vi "read_avg_traj_pks.vi"(0 "all rows":dbl[][](array[numeric])) -> (4 "Graph":cluster{"Locations":dbl[], "Amplitudes":dbl[]}[](graph), 5 "avg_trajx":dbl[](array[numeric]), 6 "avg_trajy":dbl[](array[numeric]), 7 "avg_trajz":dbl[](array[numeric]), 8 "std_trajz":dbl, 9 "std_trajx":dbl, 10 "std_trajy":dbl)   [LabVIEW 2024]
uses:
  <vilib>/Analysis/NI_AALBase.lvlib
  <vilib>/Analysis/baseanly.llb/Mean (DBL).vi
  <vilib>/Analysis/NI_AAL_SigProc.lvlib
  <vilib>/Analysis/3filter.llb/Butterworth Filter (DBL).vi
panel:
  out "max value":dbl
  out "min value":dbl
  out "subarray":dbl[](array[numeric])
  out "Graph  2":cluster{"avg_trajx":dbl[], "avg_trajz":dbl[]}(graph)
  out "pkavgloctn":dbl[](array[numeric])
  out "largerv":dbl[](array[numeric])
  out "smallerv":dbl[](array[numeric])
  out "locations":i32[](array[numeric])
  out "# found y":i32
  out "# found z":i32
  out "ypkLocations":dbl[](array[numeric])
  out "zpkLocations":dbl[](array[numeric])
  out "z_pelv_center":dbl[](array[numeric])
  out "y_pelv_center":dbl[](array[numeric])
  out "x_pelv_center":dbl[](array[numeric])
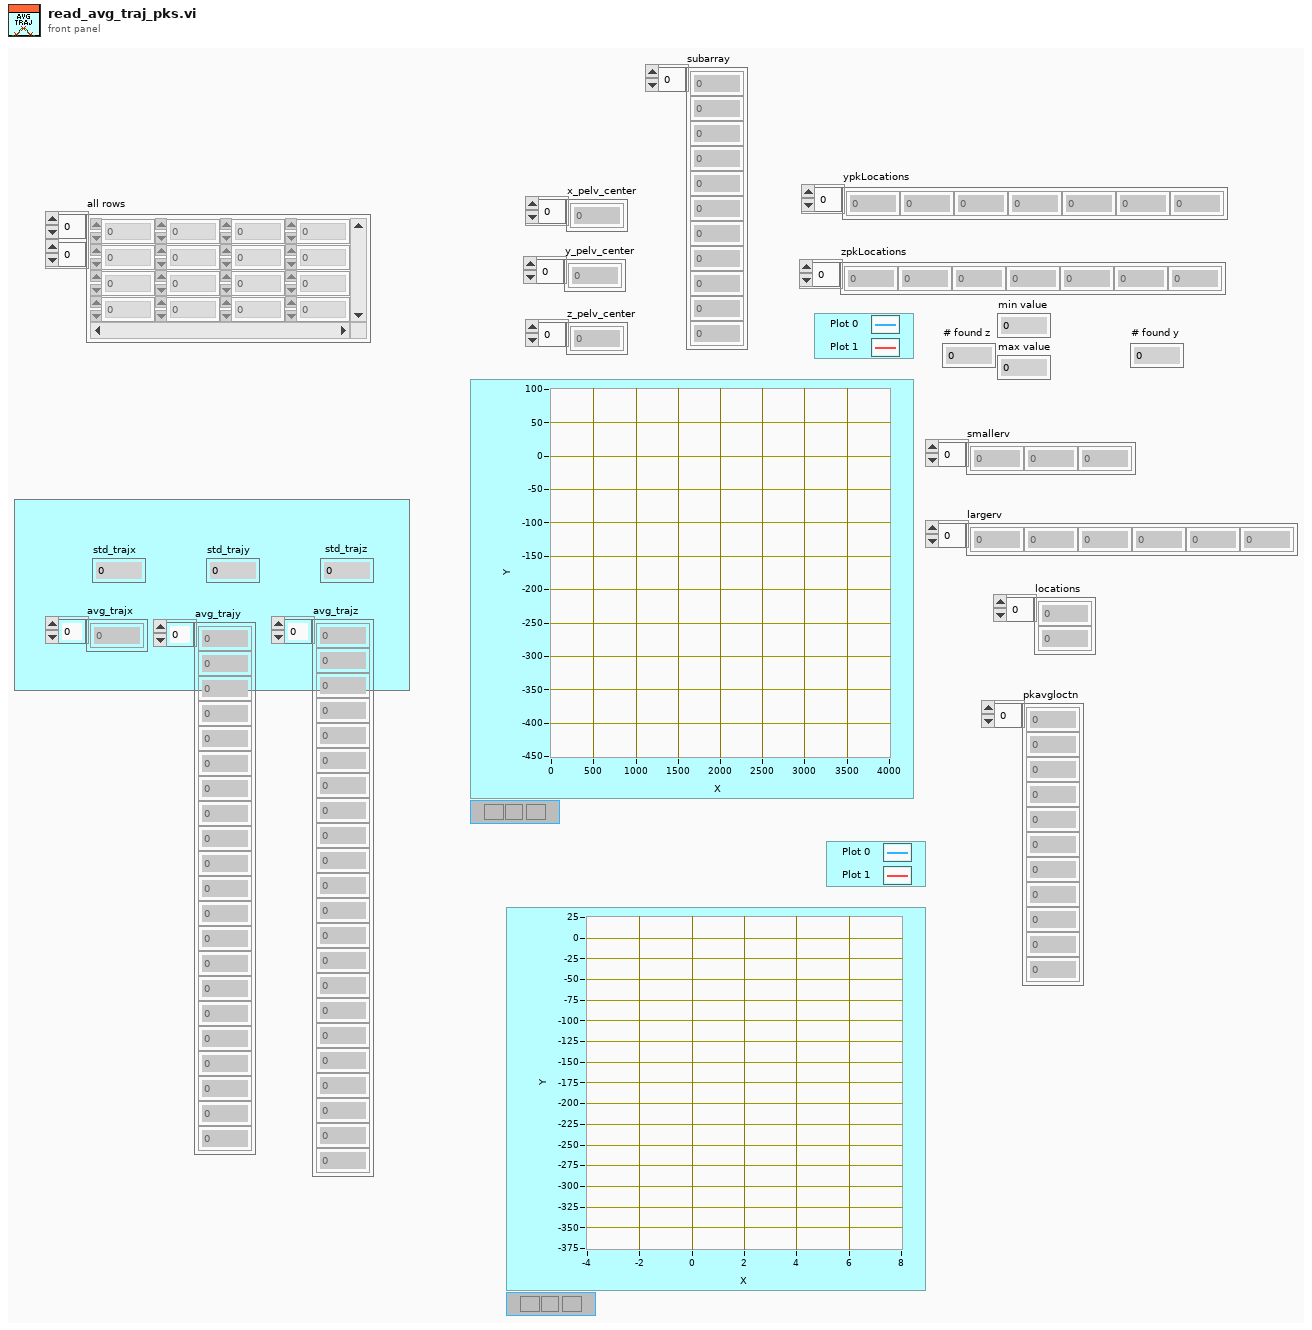
[diagram p1: front panel]
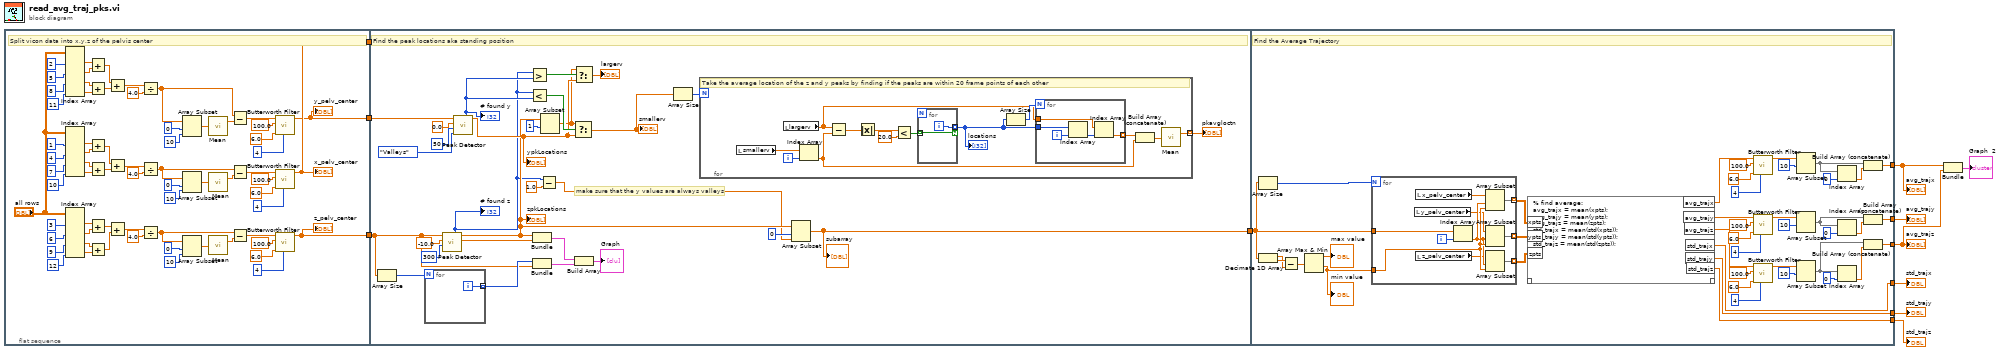
[diagram p0: block diagram]
diagram:
  n1 = flat-sequence {
    tunnel: [w12] -> w11
    tunnel: [w13] -> w10
    tunnel: [w14] -> w9
    tunnel: w11 -> [w80]
    tunnel: w10 -> [w79]
    tunnel: w9 -> [_]
    tunnel: [w81] -> w1
    tunnel: [w134] -> w5
    tunnel: [w137] -> w3
    tunnel: [w162] -> w8
    tunnel: [w129] -> w2
    tunnel: [w161] -> w7
    tunnel: [w160] -> w6
    tunnel: w1 -> [w166]
    frame #0 {
      # "Split vicon data into x,y,z of the pelvis center"
      n2 = Index Array(array="all rows", index (col) #1=2 ("disabled index (col)"), index (col) #2=5 ("index (col)"), index (col) #3=8 ("index (col)"), index (col) #4=11 ("index (col)")) -> (element #1=w59:dbl[], element #2=w58:dbl[], element #3=w57:dbl[], element #4=w56:dbl[])  [unwired: 4 in]
      n3 = Index Array(array="all rows", index (col) #1=1 ("disabled index (col)"), index (col) #2=4 ("index (col)"), index (col) #3=7 ("index (col)"), index (col) #4=10 ("index (col)")) -> (element #1=w72:dbl[], element #2=w71:dbl[], element #3=w70:dbl[], element #4=w69:dbl[])  [unwired: 4 in]
      n4 = Index Array(array="all rows", index (col) #1=3 ("disabled index (col)"), index (col) #2=6 ("index (col)"), index (col) #3=9 ("index (col)"), index (col) #4=12 ("index (col)")) -> (element #1=w46:dbl[], element #2=w45:dbl[], element #3=w44:dbl[], element #4=w43:dbl[])  [unwired: 4 in]
      n5 = Add(x=w59, y=w58) -> (x+y=w61:dbl[])
      n6 = Add(x=w57, y=w56) -> (x+y=w60:dbl[])
      n7 = Add(x=w72, y=w71) -> (x+y=w74:dbl[])
      n8 = Add(x=w70, y=w69) -> (x+y=w73:dbl[])
      n9 = Add(x=w46, y=w45) -> (x+y=w48:dbl[])
      n10 = Add(x=w44, y=w43) -> (x+y=w47:dbl[])
      n11 = Add(x=w61, y=w60) -> (x+y=w54:dbl[])
      n12 = Add(x=w74, y=w73) -> (x+y=w67:dbl[])
      n13 = Add(x=w48, y=w47) -> (x+y=w41:dbl[])
      n14 = Divide(x=w54, y=4.0) -> (x/y=w32:dbl[])
      n15 = Divide(x=w67, y=4.0) -> (x/y=w38:dbl[])
      n16 = Divide(x=w41, y=4.0) -> (x/y=w27:dbl[])
      n17 = Array Subset(array=w32, index=0, length=10) -> (w31:dbl[])
      n18 = Array Subset(array=w38, index=0, length=10) -> (w35:dbl[])
      n19 = Array Subset(array=w27, index=0, length=10) -> (w28:dbl[])
      n20 = call-poly <vilib>:"Mean.vi"("X"=w31) -> ("mean"=w53:dbl)  [unwired: 1 out]
      n21 = call-poly <vilib>:"Mean.vi"("X"=w35) -> ("mean"=w66:dbl)  [unwired: 1 out]
      n22 = call-poly <vilib>:"Mean.vi"("X"=w28) -> ("mean"=w40:dbl)  [unwired: 1 out]
      n23 = Subtract(x=w32, y=w53) -> (x-y=w15:dbl[])
      n24 = Subtract(x=w38, y=w66) -> (x-y=w19:dbl[])
      n25 = Subtract(x=w27, y=w40) -> (x-y=w26:dbl[])
      n26 = call-poly <vilib>:"Butterworth Filter.vi"("order"=4, "low cutoff freq: fl"=6.0, "sampling freq: fs"=100.0, "X"=w15) -> ("Filtered X"=w12:dbl[])  [unwired: 4 in, 1 out]
      "y_pelv_center" <- w12
      n27 = call-poly <vilib>:"Butterworth Filter.vi"("order"=4, "low cutoff freq: fl"=6.0, "sampling freq: fs"=100.0, "X"=w19) -> ("Filtered X"=w14:dbl[])  [unwired: 4 in, 1 out]
      "x_pelv_center" <- w14
      n28 = call-poly <vilib>:"Butterworth Filter.vi"("order"=4, "low cutoff freq: fl"=6.0, "sampling freq: fs"=100.0, "X"=w26) -> ("Filtered X"=w13:dbl[])  [unwired: 4 in, 1 out]
      "z_pelv_center" <- w13
    }
    frame #1 {
      # "make sure that the y values are always valleys"
      # "Find the peak locations aka standing position"
      n29 = Array Size(array=w79) -> (size(s)=w105:i32)
      n30 = for {
        N: w105 -> [_]
        tunnel: [w128] -> w101 mode=indexing
        i -> [w128]
      }
      n31 = call <vilib>:"Peak Detector.vi"("width"=300, "threshold"=-10.0, "X"=w79) -> ("Amplitudes"=w106:dbl[], "Locations"=w86:dbl[], "# found"=w83:i32)  [unwired: 4 in, 2 out]
      "zpkLocations" <- w86
      "# found z" <- w83
      n32 = call <vilib>:"Peak Detector.vi"("peaks/valleys"=enum32{"Peaks", "Valleys"}."Valleys", "width"=50, "threshold"=0.0, "X"=w80) -> ("Locations"=w95:dbl[], "# found"=w97:i32)  [unwired: 3 in, 3 out]
      "ypkLocations" <- w95
      "# found y" <- w97
      n33 = Greater?(x=w83, y=w97) -> (0:w96:bool)
      n34 = Less?(x=w83, y=w97) -> (x < y?=w98:bool)
      n35 = Bundle("Locations"=w86, "Amplitudes"=w106) -> (w104:cluster{"Locations":dbl[], "Amplitudes":dbl[]})  [unwired: 1 in]
      n36 = Bundle(w101, "Filtered X"=w79) -> (w102:cluster{i32[], "Filtered X":dbl[]})  [unwired: 1 in]
      n37 = Subtract(x=w83, y=1.0) -> (x-y=w82:dbl)
      n38 = Array Subset(array=w86, index=1) -> (w88:dbl[])  [unwired: 1 in]
      n39 = Select(t=w88, s=w98, f=w95) -> (s? t:f=w94:dbl[])
      "smallerv" <- w94
      n40 = Select(t=w88, s=w96, f=w95) -> (s? t:f=→"largerv":dbl[])
      n41 = Build Array(w104, w102) -> (→"Graph":cluster{"Locations":dbl[], "Filtered X":dbl[]}[])
      n42 = Array Size(array=w94) -> (size(s)=w92:i32)
      n43 = for {
        N: w92 -> [_]
        tunnel: [w108] -> w87 mode=indexing
        i -> [w120]
        # "Take the average location of the z and y peaks by finding if the peaks are within 20 frame points of each other"
        n44 = local read "smallerv"() -> (w119:dbl[])
        n45 = local read "largerv"() -> (w113:dbl[])
        n46 = Index Array(array=w119, index=w120) -> (element=w110:dbl)
        n47 = Subtract(x=w113, y=w110) -> (x-y=w116:dbl[])
        n48 = Absolute Value(x=w116) -> (abs(x)=w117:dbl[])
        n49 = Less?(x=w117, y=20.0) -> (x < y?=w118:bool[])
        n50 = for {
          tunnel: w118 -> [w127] mode=indexing
          tunnel: [w126] -> w112 mode=indexing if=w127
          i -> [w126]
        }
        "locations" <- w112
        n51 = Array Size(array=w112) -> (size(s)=w114:i32)
        n52 = for {
          N: w114 -> [_]
          tunnel: w113 -> [w125]
          tunnel: w112 -> [w123]
          tunnel: [w121] -> w111 mode=indexing
          i -> [w124]
          n53 = Index Array(array=w123, index=w124) -> (element=w122:i32)
          n54 = Index Array(array=w125, index=w122) -> (element=w121:dbl)
        }
        n55 = Build Array (concatenate)(w111, w110) -> (w109:dbl[])
        n56 = call-poly <vilib>:"Mean.vi"("X"=w109) -> ("mean"=w108:dbl)  [unwired: 1 out]
      }
      "pkavgloctn" <- w87
      n57 = Array Subset(array=w86, index=0, length=w82) -> (w81:dbl[])
      "subarray" <- w81
    }
    frame #2 {
      # "Find the Average Trajectory"
      n58 = Array Size(array=w166) -> (size(s)=w168:i32)
      n59 = Decimate 1D Array(w166) -> (w170:dbl[], w171:dbl[])
      n60 = Subtract(x=w171, y=w170) -> (x-y=w169:dbl[])
      n61 = Array Max & Min(array=w169) -> (max value=→"max value":dbl, min value=w167:dbl)  [unwired: 2 out]
      "min value" <- w167
      n62 = for {
        N: w168 -> [_]
        tunnel: w167 -> [w181]
        tunnel: w166 -> [w180]
        tunnel: [w174] -> w165 mode=indexing
        tunnel: [w173] -> w164 mode=indexing
        tunnel: [w172] -> w163 mode=indexing
        i -> [w179]
        n63 = local read "y_pelv_center"() -> (w176:dbl[])
        n64 = local read "x_pelv_center"() -> (w177:dbl[])
        n65 = local read "z_pelv_center"() -> (w175:dbl[])
        n66 = Index Array(array=w180, index=w179) -> (element=w178:dbl)
        n67 = Array Subset(array=w177, index=w178, length=w181) -> (w174:dbl[])
        n68 = Array Subset(array=w176, index=w178, length=w181) -> (w173:dbl[])
        n69 = Array Subset(array=w175, index=w178, length=w181) -> (w172:dbl[])
      }
      n70 = mathscript code="% find average:\navg_trajx = mean(xpts);\navg_trajy = mean(ypts);\navg_trajz = mean(zpts);\nstd_trajx = mean(std(xpts));\nstd_trajy = mean(std(ypts));\nstd_trajz = mean(std(zpts));"("xpts"=w165, "ypts"=w164, "zpts"=w163) -> ("avg_trajx"=w156:dbl[], "avg_trajy"=w152:dbl[], "avg_trajz"=w148:dbl[], "std_trajx"=w160:dbl, "std_trajy"=w162:dbl, "std_trajz"=w161:dbl)  [unwired: 1 in, 1 out]
      n71 = call-poly <vilib>:"Butterworth Filter.vi"("order"=4, "low cutoff freq: fl"=6.0, "sampling freq: fs"=100.0, "X"=w156) -> ("Filtered X"=w146:dbl[])  [unwired: 4 in, 1 out]
      n72 = call-poly <vilib>:"Butterworth Filter.vi"("order"=4, "low cutoff freq: fl"=6.0, "sampling freq: fs"=100.0, "X"=w152) -> ("Filtered X"=w144:dbl[])  [unwired: 4 in, 1 out]
      n73 = call-poly <vilib>:"Butterworth Filter.vi"("order"=4, "low cutoff freq: fl"=6.0, "sampling freq: fs"=100.0, "X"=w148) -> ("Filtered X"=w142:dbl[])  [unwired: 4 in, 1 out]
      n74 = Array Subset(array=w146, index=10) -> (w139:dbl[])  [unwired: 1 in]
      n75 = Array Subset(array=w144, index=10) -> (w133:dbl[])  [unwired: 1 in]
      n76 = Array Subset(array=w142, index=10) -> (w130:dbl[])  [unwired: 1 in]
      n77 = Index Array(array=w139, index=0) -> (element=w138:dbl)
      n78 = Index Array(array=w133, index=0) -> (element=w135:dbl)
      n79 = Index Array(array=w130, index=0) -> (element=w131:dbl)
      n80 = Build Array (concatenate)(w139, w138) -> (w137:dbl[])
      n81 = Build Array (concatenate)(w133, w135) -> (w134:dbl[])
      n82 = Build Array (concatenate)(w130, w131) -> (w129:dbl[])
    }
  }
  n83 = Bundle(w3, w2) -> (→"Graph  2":cluster{dbl[], dbl[]})  [unwired: 1 in]
  "avg_trajy" <- w5
  "avg_trajx" <- w3
  "std_trajy" <- w8
  "avg_trajz" <- w2
  "std_trajz" <- w7
  "std_trajx" <- w6
